vi "DPID.FG.vi"(7 "Action":T1, 8 "error in (no error)":errorcluster, 10 "DPID":T2, 11 "Device Item Ref in":T4 format="%.0x") -> (0 "error out":errorcluster, 2 "DPID":T2, 3 "Device Item Ref out":T4=18446744073709551615 format="%.0x")   [LabVIEW 2015, in "Diagnostics Addon System Explorer.lvlib"]
uses:
  Diagnostics Addon System Explorer.lvlib
  <vilib>/NI Veristand/Custom Device API/Custom Device Item Ref.ctl
  Shared/Types/DPID.ctl
  Shared/Types/DPID.Rate.ctl
  Types/FG.Action.ctl
  <vilib>/NI Veristand/Custom Device API/Get Item Property (U32 Array).vi
  <vilib>/NI Veristand/Custom Device API/Get Item Property (U32).vi
  <vilib>/NI/NI VeriStand Advanced SysDef API/_SubVIs/SysDef.Property.Set.U32.vi
  Shared/SubVIs/Constants.vi
  <vilib>/NI/NI VeriStand Advanced SysDef API/_SubVIs/SysDef.Property.Set.U32.Array.vi
  Shared/Diagnostics Addon Shared.lvlib
  <vilib>/NI VeriStand/Custom Device API/Custom Device API.lvlib
  <vilib>/NI/NI VeriStand Advanced SysDef API/SysDef API/Advanced System Definition.lvlib
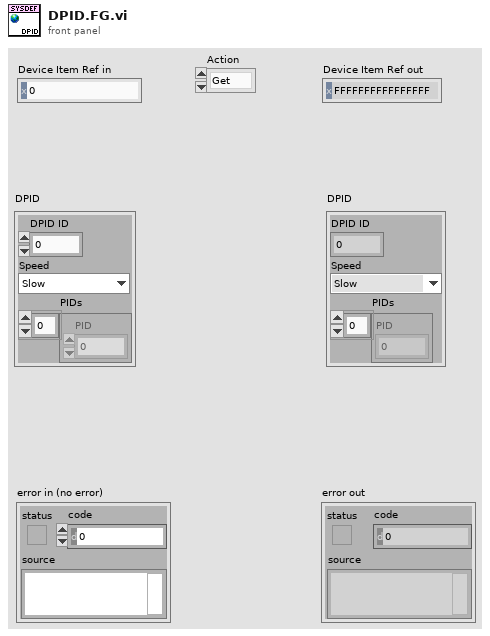
[diagram p1: front panel]
types:
  T1 = typedef "Diagnostics Addon System Explorer.lvlib/FG.Action.ctl" = enum16{"Get", "Set"}
  T2 = typedef "Diagnostics Addon Shared.lvlib/DPID.ctl" = cluster{"DPID ID":u8, "Speed":T3, "PIDs":u16[]}
  T3 = typedef "Diagnostics Addon Shared.lvlib/DPID.Rate.ctl" = enum16{"Slow", "Medium", "Fast"}
  T4 = typedef "Custom Device API.lvlib/Custom Device Item Ref.ctl" = u64
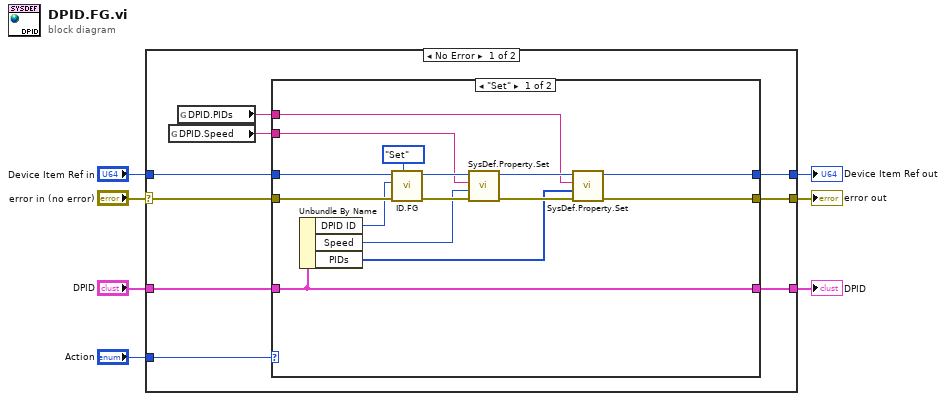
[diagram p0: block diagram]
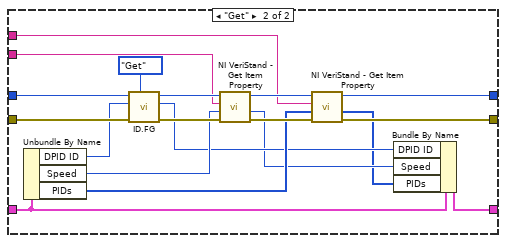
[diagram p2: hidden frame]
diagram:
  n1 = case shown="No Error" "error in (no error)" {
    selector: "error in (no error)" -> [w16 w51]
    tunnel: "Device Item Ref in" -> [w15 w52]
    tunnel: [w14 w52] -> w4
    tunnel: [w13 w51] -> w5
    tunnel: [w12 _] -> w3
    tunnel: "DPID" -> [w11 _]
    tunnel: "Action" -> [w10 _]
    frame No Error {
      n2 = global read "Constants.vi" "DPID.Speed"() -> (w9:string)
      n3 = global read "Constants.vi" "DPID.PIDs"() -> (w8:string)
      n4 = case shown="\"Set\"" w10 {
        tunnel: w16 -> [w29 w50]
        tunnel: w15 -> [w30 w49]
        tunnel: [w21 w38] -> w14
        tunnel: [w22 w37] -> w13
        tunnel: [w31 w32] -> w12
        tunnel: w11 -> [w31 w36]
        tunnel: w9 -> [w19 w45]
        tunnel: w8 -> [w18 w39]
        frame "Set" {
          n5 = Unbundle By Name(w31) -> ("DPID ID"=w27:u8, "Speed"=w20:T3, "PIDs"=w17:u16[])
          n6 = call "ID.FG.vi"("Action"=FG.Action."Set", "error in (no error)"=w29, "ID"=w27, "Device Item Ref in"=w30) -> ("error out"=w24:errorcluster, "Device Item Ref out"=w23:T4)  [unwired: 5 in, 1 out]
          n7 = call-poly <vilib>:"SysDef.Property.Set.vi"("error in (no error)"=w24, "Value"=w20, "Property Name"=w19, "nodeID"=w23) -> ("error out"=w26:errorcluster, "nodeID out"=w25:u64)  [unwired: 6 in]
          n8 = call-poly <vilib>:"SysDef.Property.Set.vi"("error in (no error)"=w26, "Value"=w17, "Property Name"=w18, "nodeID"=w25) -> ("error out"=w22:errorcluster, "nodeID out"=w21:u64)  [unwired: 6 in]
        }
        frame "Get" {
          n9 = Unbundle By Name(w36) -> ("DPID ID"=w44:u8, "Speed"=w43:T3, "PIDs"=w40:u16[])
          n10 = call "ID.FG.vi"("Action"=FG.Action."Get", "error in (no error)"=w50, "ID"=w44, "Device Item Ref in"=w49) -> ("error out"=w46:errorcluster, "ID"=w35:u32, "Device Item Ref out"=w48:T4)  [unwired: 5 in]
          n11 = call-poly <vilib>:"NI VeriStand - Get Item Property.vi"("error in (no error)"=w46, "Default Value"=w43, "Property Name"=w45, "Item Ref in"=w48) -> ("error out"=w42:errorcluster, "Value"=w34:u32, "Item Ref out"=w41:T4)  [unwired: 4 in, 1 out]
          n12 = call-poly <vilib>:"NI VeriStand - Get Item Property.vi"("error in (no error)"=w42, "Default Value"=w40, "Property Name"=w39, "Item Ref in"=w41) -> ("error out"=w37:errorcluster, "Value"=w33:u32[], "Item Ref out"=w38:T4)  [unwired: 4 in, 1 out]
          n13 = Bundle By Name(cluster=w36, "DPID ID"=w35, "Speed"=w34, "PIDs"=w33) -> (w32:T2)
        }
      }
    }
    frame Error {
    }
  }
  "error out" <- w5
  "Device Item Ref out" <- w4
  "DPID" <- w3
